vi "Untitled 1.vi"   [LabVIEW 2020]
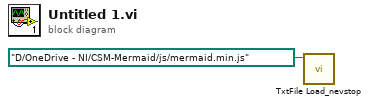
[diagram p0: block diagram]
diagram:
  n1 = call <userlib>:"TxtFile Load_nevstop.vi"("Path"=path "D:/OneDrive - NI/CSM-Mermaid/js/mermaid.min.js") -> ()  [unwired: 9 in, 2 out]
